vi "_Get Parameter List.vi"(4 "error in (no error)":errorcluster, 6 "Parameter Type":T1=enum."Experiment Parameters", 7 "node in":refnum<k20>) -> (0 "error out":errorcluster, 2 "Parameters List":string[][](array[string]), 3 "node out":refnum<k20>)   [LabVIEW 2015]
uses:
  Server/AutoCal/Controls/xml Parameter Type.ctl
  <vilib>/xml/Close Reference(Node).vi
  <vilib>/xml/NI_XML.lvlib
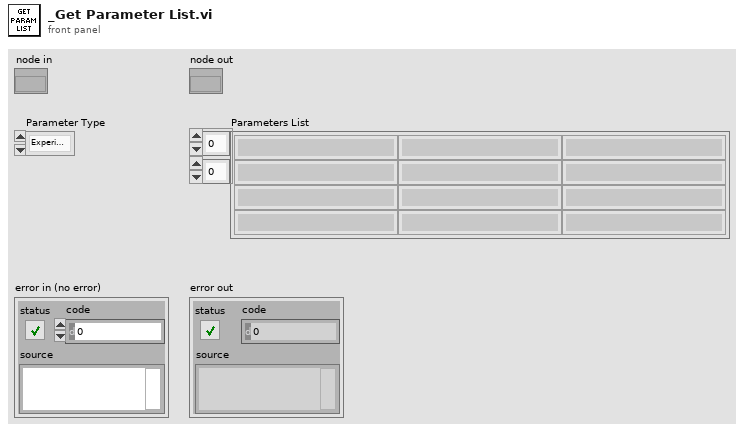
[diagram p1: front panel]
types:
  T1 = typedef "xml Parameter Type.ctl" = enum16{"Method Parameters", "Experiment Parameters"}
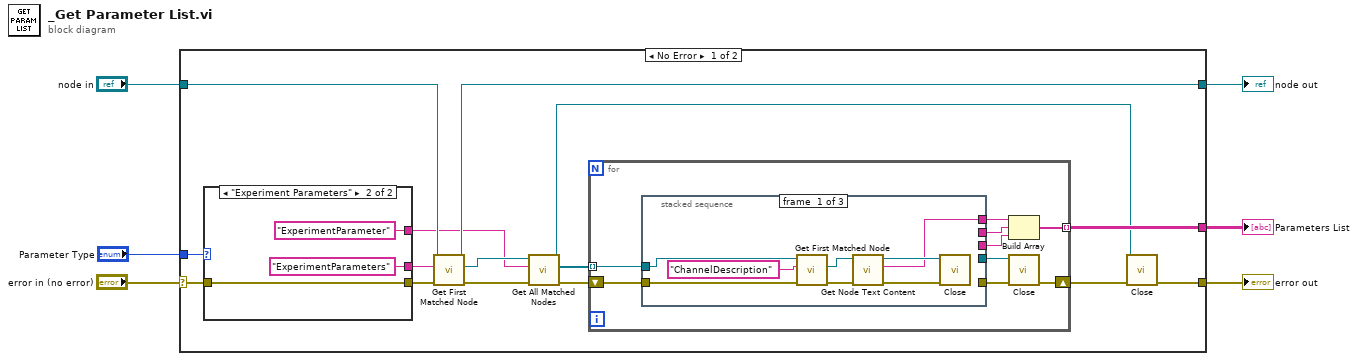
[diagram p0: block diagram]
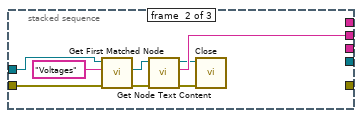
[diagram p2: hidden frame]
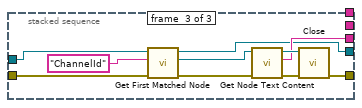
[diagram p3: hidden frame]
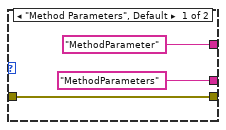
[diagram p4: hidden frame]
diagram:
  n1 = case shown="No Error" "error in (no error)" {
    selector: "error in (no error)" -> [w9 w63]
    tunnel: [w19 _] -> w6
    tunnel: "node in" -> [w18 w64]
    tunnel: [w17 w64] -> w3
    tunnel: [w12 w63] -> w2
    tunnel: "Parameter Type" -> [w11 _]
    frame No Error {
      n2 = case shown="\"Experiment Parameters\"" w11 {
        tunnel: [w59 w62] -> w10
        tunnel: w9 -> [w59 w62]
        tunnel: ["MethodParameters" ("XPath expression") "ExperimentParameters" ("XPath expression")] -> w8
        tunnel: ["MethodParameter" ("XPath expression") "ExperimentParameter" ("XPath expression")] -> w7
        frame "Method Parameters", Default {
        }
        frame "Experiment Parameters" {
        }
      }
      n3 = call <vilib>:"Get First Matched Node.vi"("error in (no error)"=w10, "XPath expression"=w8, "node in"=w18) -> ("error out"=w15:errorcluster, "node result"=w16:refnum<k20>, "node out"=w17:refnum<k20>)  [unwired: 6 in]
      n4 = call <vilib>:"Get All Matched Nodes.vi"("error in (no error)"=w15, "XPath expression"=w7, "node in"=w16) -> ("error out"=w21:errorcluster, "node result array"=w20:refnum<k20>[], "node out"=w13:refnum<k20>)  [unwired: 6 in]
      n5 = for {
        shift-right: [w28] -> w14
        shift-left: w21 -> [w29]
        tunnel: w20 -> [w30] mode=indexing
        tunnel: [w24] -> w19 mode=indexing
        n6 = stacked-sequence {
          tunnel: w30 -> [w38 w46 w56]
          tunnel: w29 -> [w37 w45 w55]
          tunnel: [w31 _ _] -> w27
          tunnel: [_ w42 _] -> w26
          tunnel: [_ _ w50] -> w25
          tunnel: [_ _ w49] -> w23
          tunnel: [_ _ w48] -> w22
          frame #0 {
            n7 = call <vilib>:"Get First Matched Node.vi"("error in (no error)"=w37, "XPath expression"="ChannelDescription", "node in"=w38) -> ("error out"=w34:errorcluster, "node result"=w35:refnum<k20>)  [unwired: 6 in, 1 out]
            n8 = call <vilib>:"Get Node Text Content.vi"("error in (no error)"=w34, "node in"=w35) -> ("error out"=w32:errorcluster, "node text"=w31:string, "node out"=w33:refnum<k20>)  [unwired: 7 in]
            n9 = call-poly <vilib>:"Close.vi"("error in (no error)"=w32, "node"=w33) -> ()  [unwired: 7 in, 1 out]
          }
          frame #1 {
            n10 = call <vilib>:"Get First Matched Node.vi"("error in (no error)"=w45, "XPath expression"="Voltages", "node in"=w46) -> ("error out"=w39:errorcluster, "node result"=w43:refnum<k20>)  [unwired: 6 in, 1 out]
            n11 = call <vilib>:"Get Node Text Content.vi"("error in (no error)"=w39, "node in"=w43) -> ("error out"=w40:errorcluster, "node text"=w42:string, "node out"=w41:refnum<k20>)  [unwired: 7 in]
            n12 = call-poly <vilib>:"Close.vi"("error in (no error)"=w40, "node"=w41) -> ()  [unwired: 7 in, 1 out]
          }
          frame #2 {
            n13 = call <vilib>:"Get First Matched Node.vi"("error in (no error)"=w55, "XPath expression"="ChannelId", "node in"=w56) -> ("error out"=w53:errorcluster, "node result"=w54:refnum<k20>, "node out"=w49:refnum<k20>)  [unwired: 6 in]
            n14 = call <vilib>:"Get Node Text Content.vi"("error in (no error)"=w53, "node in"=w54) -> ("error out"=w52:errorcluster, "node text"=w50:string, "node out"=w51:refnum<k20>)  [unwired: 7 in]
            n15 = call-poly <vilib>:"Close.vi"("error in (no error)"=w52, "node"=w51) -> ("error out"=w48:errorcluster)  [unwired: 7 in]
          }
        }
        n16 = Build Array(w27, w26, w25) -> (w24:string[])
        n17 = call-poly <vilib>:"Close.vi"("error in (no error)"=w22, "node"=w23) -> ("error out"=w28:errorcluster)  [unwired: 7 in]
      }
      n18 = call-poly <vilib>:"Close.vi"("error in (no error)"=w14, "node"=w13) -> ("error out"=w12:errorcluster)  [unwired: 7 in]
    }
    frame Error {
    }
  }
  "Parameters List" <- w6
  "error out" <- w2
  "node out" <- w3
